vi "Get String.vi"(5 "use temporary file? (F)":bool, 7 "data type of variable":string, 8 "error in":errorcluster, 10 "variable name":string, 11 "GOLPI ref. in":T1={"pipe handle"={"lv_proc.dll file path"=path "", "process instance handle"=[], "debug mode"=FALSE, "debug data"=[]}, "fast read timeout [ms]"=500, "fast read settle time [ms]"=10, "fast read to multiple [ms]"=1, "max elements per input line"=100, "slow read timeout [ms]"=5000, "stdin double format specifier"="%_16e", "max elements per stdout output column"=100, "console mode bitstream"=FALSE, "bitstream first read timeout [ms]"=1000, "bitstream read timeout [ms]"=50, "struct transfer possible"=FALSE, "matlab mode"=FALSE}) -> (0 "error out":errorcluster, 2 "value":string, 3 "GOLPI ref. out":T1={"pipe handle"={"lv_proc.dll file path"=path "", "process instance handle"=[], "debug mode"=FALSE, "debug data"=[]}, "fast read timeout [ms]"=500, "fast read settle time [ms]"=10, "fast read to multiple [ms]"=1, "max elements per input line"=100, "slow read timeout [ms]"=5000, "stdin double format specifier"="%_16e", "max elements per stdout output column"=100, "console mode bitstream"=FALSE, "bitstream first read timeout [ms]"=1000, "bitstream read timeout [ms]"=50, "struct transfer possible"=FALSE, "matlab mode"=FALSE})   [LabVIEW 2020, in "GOLPI library.lvlib"]
doc: "Part of polymorph Get Variable.vi"
uses:
  GOLPI library.lvlib
  GOLPI reference Type Def.ctl
  Pipe Handle.ctl
  Bitstream Data Type.ctl
  Custom Error Codes Enum Type Def.vi
  LV Process library.lvlib
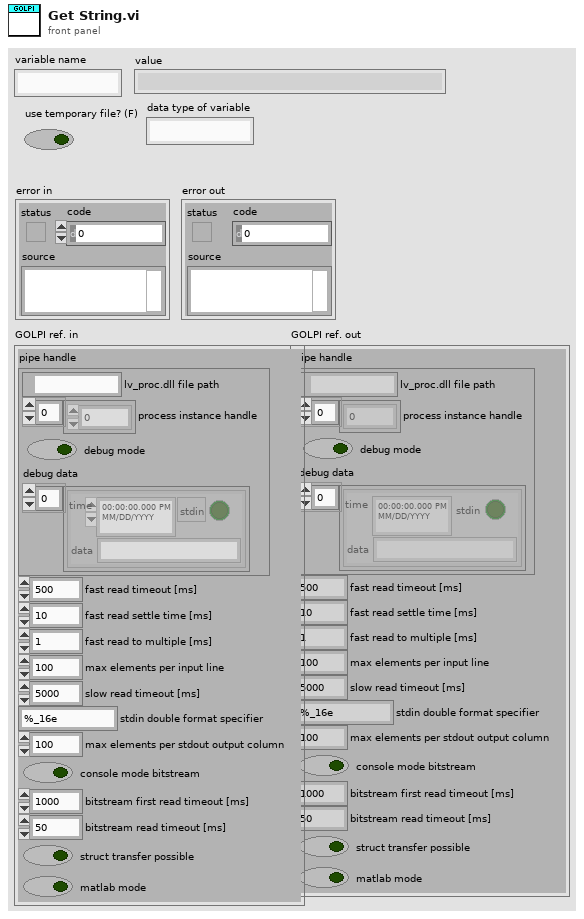
[diagram p1: front panel]
types:
  T1 = typedef "GOLPI library.lvlib/GOLPI reference Type Def.ctl" = cluster{"pipe handle":T2, "fast read timeout [ms]":u32, "fast read settle time [ms]":u32, "fast read to multiple [ms]":u32, "max elements per input line":u32, "slow read timeout [ms]":u32, "stdin double format specifier":string, "max elements per stdout output column":u32, "console mode bitstream":bool, "bitstream first read timeout [ms]":u32, "bitstream read timeout [ms]":u32, "struct transfer possible":bool, "matlab mode":bool}
  T2 = typedef "LV Process library.lvlib/Pipe Handle.ctl" = cluster{"lv_proc.dll file path":path, "process instance handle":u32[], "debug mode":bool, "debug data":cluster{"time":timestamp, "stdin":bool, "data":string}[]}
  T3 = typedef "GOLPI library.lvlib/Bitstream Data Type.ctl" = enum16{"dummy", "int", "uint", "float", "complex", "str", "real numeric"}
  T4 = typedef "GOLPI library.lvlib/Custom Error Codes Enum Type Def.vi" = enum16{"no error", "00 working directory PAR1 missing", "01 octave binary PAR1 missing", "02 octave report error PAR1", "03 empty output last cmd PAR1", "04 missing temporary file PAR1", "05 pwd PAR 1 not exist", "06 oct package not installed", "07 octave default binary missing", "10 var PAR1 not string, vect", "11 var PAR1 not num, scal, ~compl", "12 var PAR1 not num, scal, compl", "13 var PAR1 not num, vect, ~compl", "14 var PAR1 not num, vect, compl", "15 var PAR1 not num, mat, ~compl", "16 var PAR1 not num, mat, ~compl", "30 read timeout", "60 bitstream transport failed", "61 bitstream decode error PAR1", "62 bitstream cannot be set", "70 struct transfer not possible", "80 struct: cluster elem. PAR1 not implem.", "81 struct: structure field PAR1 not implem.", "82 struct: size mismatch of PAR1", "83 struct: type mismatch of PAR1", "98 internal error", "99 not finished", "90 Not supported in Matlab mode", "91 Matlab variable transfer error", "92 Matlab Script Error"}
  T5 = typedef "GOLPI library.lvlib/Bitstream Data.ctl" = cluster{"double":dbl[][], "cplx double":cdb[][], "int64":i64[][], "uint64":u64[][], "str":string[], "data type":T3}
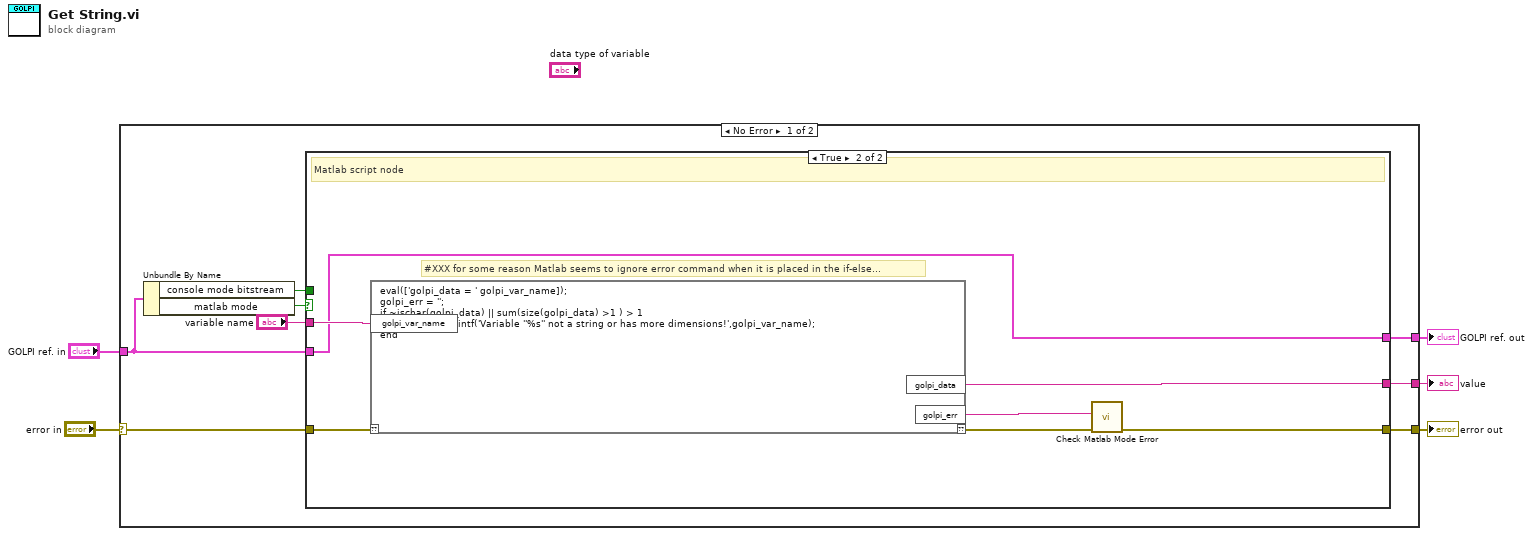
[diagram p0: block diagram]
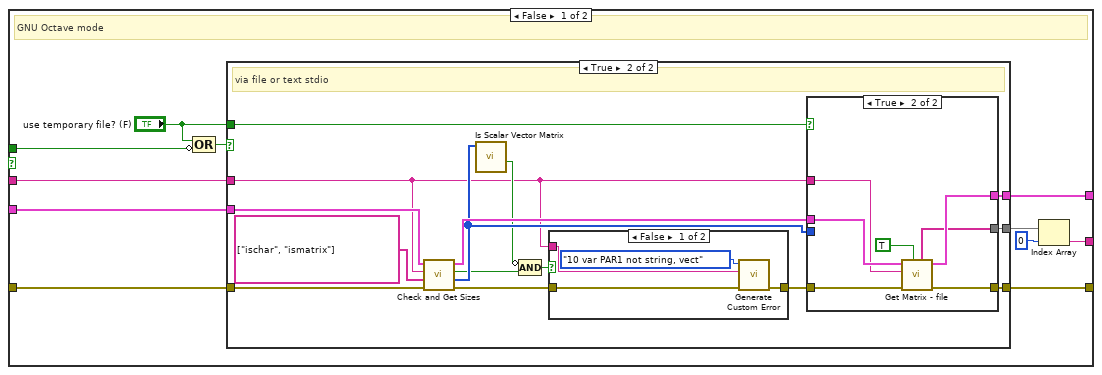
[diagram p2: hidden frame]
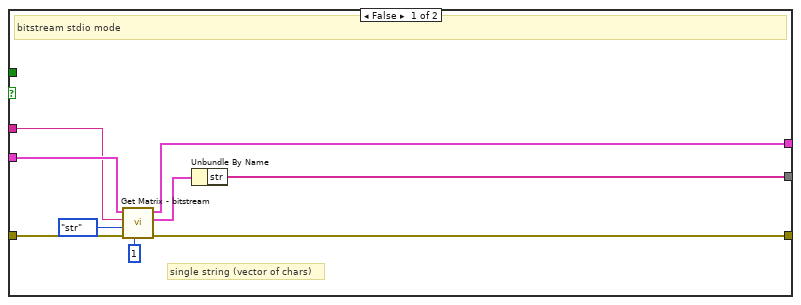
[diagram p3: hidden frame]
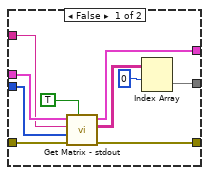
[diagram p4: hidden frame]
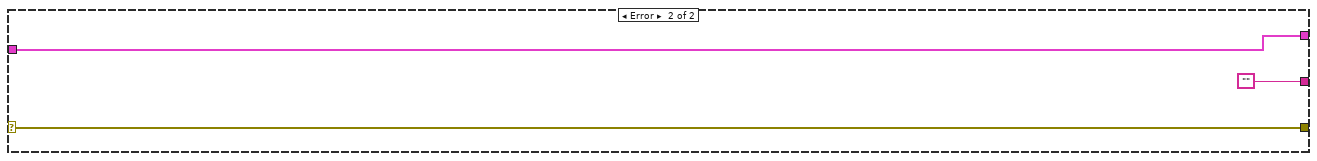
[diagram p6: hidden frame]
diagram:
  n1 = case shown="No Error" "error in" {
    selector: "error in" -> [w13 w79]
    tunnel: [w11 w79] -> w5
    tunnel: [w10 ""] -> w4
    tunnel: "GOLPI ref. in" -> [w9 w78]
    tunnel: [w12 w78] -> w1
    frame No Error {
      n2 = Unbundle By Name(w9) -> ("console mode bitstream"=w8:bool, "matlab mode"=w7:bool)
      n3 = case shown="True" w7 {
        tunnel: w13 -> [w24 w77]
        tunnel: [w23 w75] -> w12
        tunnel: [w20 w72] -> w11
        tunnel: [w19 w71] -> w10
        tunnel: w9 -> [w18 w75]
        tunnel: w8 -> [w17 _]
        tunnel: "variable name" -> [w14 w76]
        frame False {
          # "GNU Octave mode"
          n4 = Compound Arithmetic op=OR("use temporary file? (F)", invert w17) -> (w15:bool)
          n5 = case shown="True" w15 {
            tunnel: w24 -> [w33 w47]
            tunnel: w18 -> [w32 w45]
            tunnel: [w28 w42] -> w23
            tunnel: [w26 w41] -> w21
            tunnel: [w25 w40] -> w20
            tunnel: "use temporary file? (F)" -> [_ w35]
            tunnel: w14 -> [w29 w34]
            frame False {
              # "single string (vector of chars)"
              # "bitstream stdio mode"
              n6 = call "Get Matrix - bitstream.vi"("max dimensions (0: scalar)"=1, "error in (no error)"=w33, "data type"=Bitstream_Data_Type."str", "variable name"=w29, "GOLPI ref. in"=w32) -> ("error out"=w25:errorcluster, "data"=w27:T5, "GOLPI ref. out"=w28:T1)  [unwired: 4 in]
              n7 = Unbundle By Name(w27) -> ("str"=w26:string[])
            }
            frame True {
              # "via file or text stdio"
              n8 = call "Check and Get Sizes.vi"("error in (no error)"=w47, "test commands"=string[] ["ischar", "ismatrix"], "variable name"=w34, "GOLPI ref. in"=w45) -> ("error out"=w48:errorcluster, "octave sizes"=w39:i32[], "all tests OK?"=w38:bool, "GOLPI ref. out"=w43:T1)  [unwired: 4 in]
              n9 = call "Is Scalar Vector Matrix.vi"("octave sizes"=w39) -> ("is matrix?"=w36:bool)  [unwired: 5 in, 5 out]
              n10 = Compound Arithmetic op=AND(invert w36, w38) -> (w37:bool)
              n11 = case shown="False" w37 {
                tunnel: [w68 w70] -> w44
                tunnel: w48 -> [w69 w70]
                tunnel: w34 -> [w67 _]
                frame False {
                  n12 = call "Generate Custom Error.vi"("error in"=w69, "PAR1"=w67, "GOLPI error"=Custom_Error_Codes_Enum_Type_Def.vi."10 var PAR1 not string, vect" ("Enum")) -> ("error out"=w68:errorcluster)  [unwired: 8 in]
                }
                frame True {
                }
              }
              n13 = case shown="True" w35 {
                tunnel: w44 -> [w58 w65]
                tunnel: [w57 w63] -> w40
                tunnel: w43 -> [w56 w64]
                tunnel: [w55 w62] -> w42
                tunnel: w34 -> [w53 w60]
                tunnel: w39 -> [w52 _]
                tunnel: [w49 w59] -> w41
                frame False {
                  n14 = call "Get Matrix - stdout.vi"("is string?"=TRUE ("is string"), "error in (no error)"=w58, "octave sizes"=w52, "variable name"=w53, "GOLPI ref. in"=w56) -> ("error out"=w57:errorcluster, "array"=w50:string[][], "GOLPI ref. out"=w55:T1)  [unwired: 4 in]
                  n15 = Index Array(array=w50, index (row)=0) -> (element=w49:string[])  [unwired: 1 in]
                }
                frame True {
                  n16 = call "Get Matrix - file.vi"("is string?"=TRUE ("is string"), "error in (no error)"=w65, "variable name"=w60, "GOLPI ref. in"=w64) -> ("error out"=w63:errorcluster, "GOLPI ref. out"=w62:T1, "string array"=w59:string[])  [unwired: 3 in, 2 out]
                }
              }
            }
          }
          n17 = Index Array(array=w21, index=0 ("index (row)")) -> (element=w19:string)
        }
        frame True {
          # "#XXX for some reason Matlab seems to ignore error command when it is placed in the if-else..."
          # "Matlab script node"
          n18 = script code="eval(['golpi_data = ' golpi_var_name]);\ngolpi_err = '';\nif ~ischar(golpi_data) || sum(size(golpi_data) >1 ) > 1\n  golpi_err = sprintf('Variable ''%s'' not a string or has more dimensions!',golpi_var_name);\nend"("??"=w77, "golpi_var_name"=w76) -> ("??"=w74:errorcluster, "golpi_data"=w71:string, "golpi_err"=w73:string)
          n19 = call "Check Matlab Mode Error.vi"("error in"=w74, "custom error string (empty)"=w73) -> ("error out"=w72:errorcluster)  [unwired: 9 in]
        }
      }
    }
    frame Error {
    }
  }
  "value" <- w4
  "error out" <- w5
  "GOLPI ref. out" <- w1
